vi "BotPose Correction.vi"(9 "Pos In":cluster{"x":dbl, "y":dbl}={"x"=13.014915967536774, "y"=9.532980345268305}, 10 "Robot Velocities In":T3={"X Velocity"=-6.0927338461737115e-19, "Y Velocity"=3.330663501205842e-16, "Rotational \nVelocity"=-0.0823974609375}) -> (0 "BotPose":cluster{"Numeric":dbl, "Numeric":dbl}, 1 "Bordeaux Pos":cluster{dbl, dbl}, 2 "Robot Velocities Out":T3={"X Velocity"=-6.0927338461737115e-19, "Y Velocity"=3.330663501205842e-16, "Rotational \nVelocity"=-0.0823974609375})   [LabVIEW 2025]
uses:
  swerve-template/Type Definitions/Data/Robot Velocities.ctl
  Framework/Robot Global Data.vi
  <vilib>/addons/control/pid/pid.llb/PID (DBL).vi
  <vilib>/addons/control/pid/NI_PID_pid.lvlib
panel:
  in  "PID gains":T1={"proportional gain (Kc)"=2.5, "integral time (Ti, min)"=0.0, "derivative time (Td, min)"=0.0} {"derivative time (Td, min)" format="%.3f"; "integral time (Ti, min)" format="%.3f"; "proportional gain (Kc)" format="%.3f"}
  in  "output range":cluster{"output high":dbl, "output low":dbl}={"output high"=4.0, "output low"=-4.0} {"output low" format="%.2f"; "output high" format="%.2f"}
  out "Error":cluster{dbl, dbl}(graph)={-6.0927338461737115e-19, -1.21152228156357}
  out "Velocities OUT":T2(graph)={"X Velocity"=-6.0927338461737115e-19, "Y Velocity"=3.330663501205842e-16, "Rotational \nVelocity"=-0.0823974609375}
  out "Correction":cluster{dbl, dbl}(graph)={-6.0927338461737115e-19, -1.21152228156357}
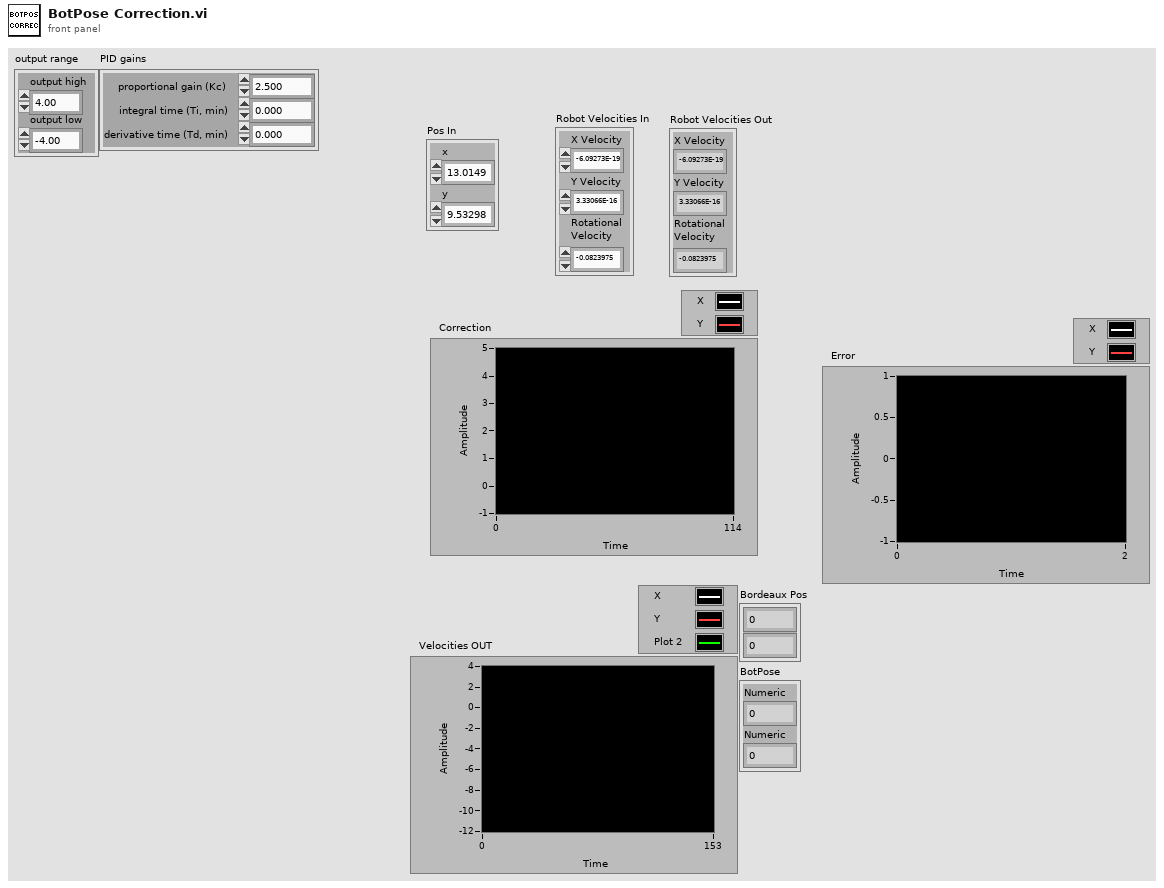
[diagram p1: front panel]
types:
  T1 = cluster{"proportional gain (Kc)":dbl, "integral time (Ti, min)":dbl, "derivative time (Td, min)":dbl}
  T2 = cluster{"X Velocity":dbl, "Y Velocity":dbl, "Rotational \nVelocity":dbl}
  T3 = typedef "Robot Velocities.ctl" = cluster{"X Velocity":dbl, "Y Velocity":dbl, "Rotational \nVelocity":dbl}
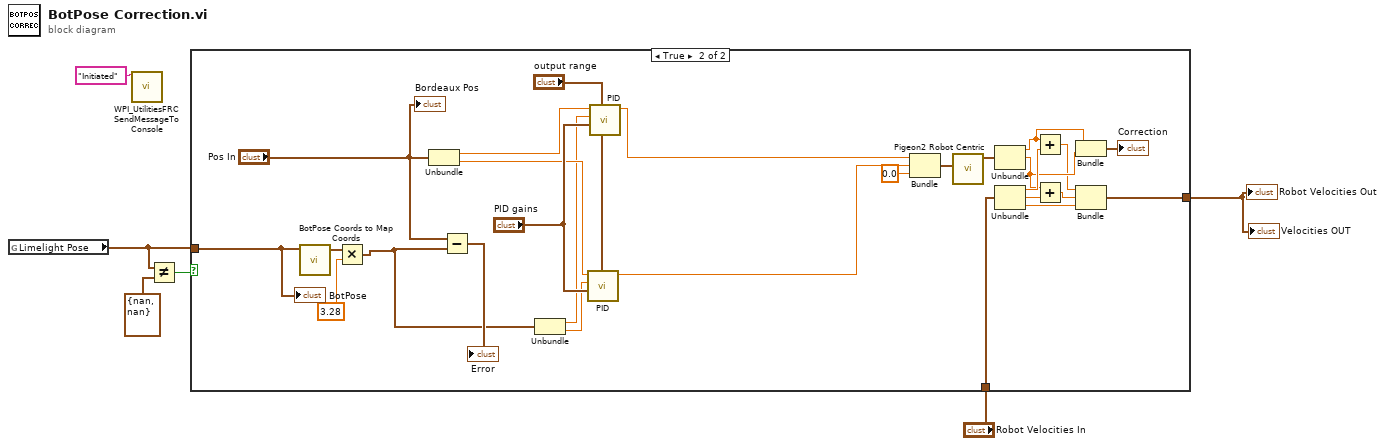
[diagram p0: block diagram]
diagram:
  n1 = global read "Robot Global Data.vi" "Limelight Pose"() -> (w3:cluster{"X":dbl, "Y":dbl})
  n2 = call <vilib>:"WPI_UtilitiesFRC SendMessageToConsole.vi"("Message"="Initiated") -> ()  [unwired: 14 in, 1 out]
  n3 = Not Equal?(x=w3, y=cluster{"X":dbl, "Y":dbl} {"X"=nan, "Y"=nan}) -> (x != y?=w1:bool)
  n4 = case shown="True" w1 {
    tunnel: w3 -> [_ w11]
    tunnel: [w7 w22] -> w5
    tunnel: "Robot Velocities In" -> [w7 w34]
    frame False {
    }
    frame True {
      n5 = call "BotPose Coords to Map Coords.vi"("Point In"=w11) -> ("Point Out"=w10:cluster{dbl, dbl})  [unwired: 10 in]
      n6 = Multiply(x=w10, y=3.28) -> (x*y=w8:cluster{dbl, dbl})
      n7 = Unbundle("Pos In") -> ("x"=w18:dbl, "y"=w17:dbl)
      n8 = Subtract(x="Pos In", y=w8) -> (x-y=→"Error":cluster{dbl, dbl})
      n9 = Unbundle(w8) -> (w16:dbl, w15:dbl)
      n10 = call-poly <vilib>:"PID.vi"("output range"="output range", "PID gains"="PID gains", "process variable"=w15, "setpoint"=w17) -> ("output"=w13:dbl)  [unwired: 6 in, 1 out]
      n11 = call-poly <vilib>:"PID.vi"("output range"="output range", "PID gains"="PID gains", "process variable"=w16, "setpoint"=w18) -> ("output"=w14:dbl)  [unwired: 6 in, 1 out]
      n12 = Bundle("output"=w14, "output"=w13, 0.0) -> (w31:cluster{"output":dbl, "output":dbl, dbl})  [unwired: 1 in]
      n13 = call "Pigeon2 Robot Centric.vi"("Robot Centric Velocities"=w31) -> ("Field Centric Velocities"=w30:T3)  [unwired: 10 in]
      n14 = Unbundle(w30) -> ("X Velocity"=w24:dbl, "Y Velocity"=w23:dbl)  [unwired: 1 out]
      n15 = Unbundle(w34) -> ("X Velocity"=w25:dbl, "Y Velocity"=w28:dbl, "Rotational \nVelocity"=w32:dbl)
      n16 = Add(x=w24, y=w25) -> (x+y=w21:dbl)
      n17 = Add(x=w23, y=w28) -> (x+y=w27:dbl)
      n18 = Bundle("X Velocity"=w24, "Y Velocity"=w23) -> (→"Correction":cluster{"X Velocity":dbl, "Y Velocity":dbl})  [unwired: 1 in]
      n19 = Bundle(w21, w27, "Rotational \nVelocity"=w32) -> (w22:cluster{dbl, dbl, "Rotational \nVelocity":dbl})  [unwired: 1 in]
      "Bordeaux Pos" <- "Pos In"
      "BotPose" <- w11
    }
  }
  "Robot Velocities Out" <- w5
  "Velocities OUT" <- w5
